vi "Signal Generator Calibration Sub VI (FINAL).vi"(1 "error in (no error)":errorcluster, 3 "VISA resource name":refnum<visa-resource-name>) -> (0 "error out":errorcluster, 2 "Confirmed Instrument Name":string)   [LabVIEW 2017]
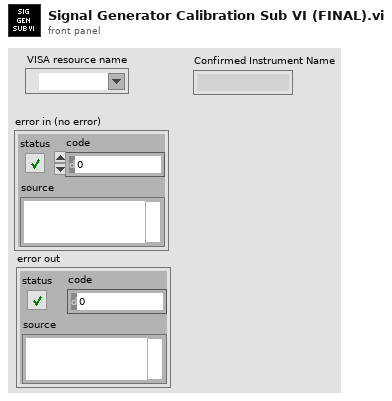
[diagram p1: front panel]
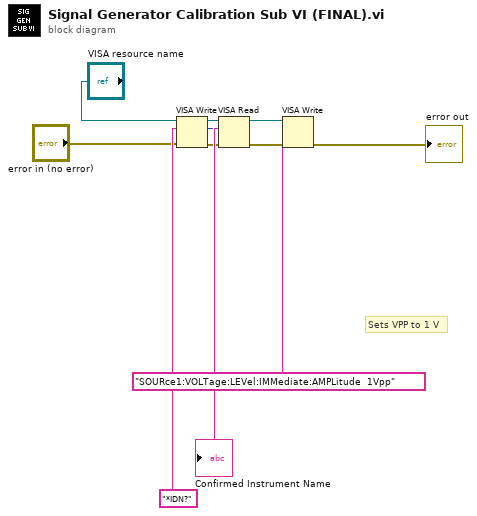
[diagram p0: block diagram]
diagram:
  # "Sets VPP to 1 V"
  n1 = VISA Write(VISA resource name="VISA resource name", write buffer="*IDN?", error in (no error)="error in (no error)") -> (VISA resource name out=w7:refnum<visa-resource-name>, return count=w8:u32, error out=w9:errorcluster)
  n2 = VISA Read(VISA resource name=w7, byte count=w8, error in (no error)=w9) -> (VISA resource name out=w2:refnum<visa-resource-name>, read buffer=→"Confirmed Instrument Name":string, error out=w4:errorcluster)  [unwired: 1 out]
  n3 = VISA Write(VISA resource name=w2, write buffer="SOURce1:VOLTage:LEVel:IMMediate:AMPLitude  1Vpp", error in (no error)=w4) -> (error out=→"error out":errorcluster)  [unwired: 2 out]
